vi "Ensure Parents are Expanded.vi"(8 "error in":errorcluster, 11 "Tree":refnum<vi>) -> (0 "error out":errorcluster)   [LabVIEW 2020]
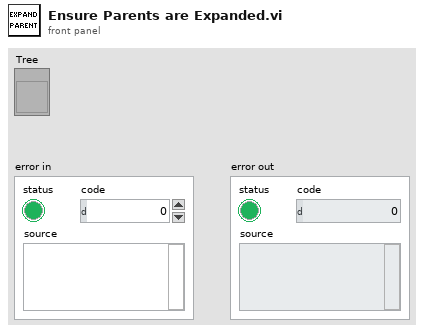
[diagram p1: front panel]
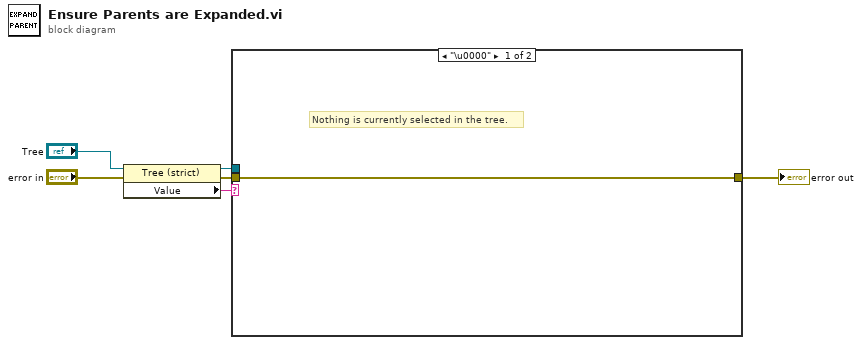
[diagram p0: block diagram]
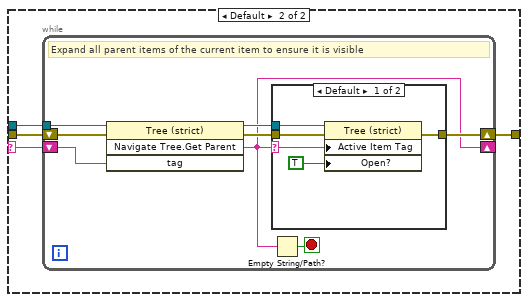
[diagram p2: hidden frame]
diagram:
  n1 = property class="Tree (strict)"(reference="Tree", error in="error in") -> (reference out=w1:refnum<vi>, error out=w5:errorcluster, "Value"=w2:string)
  n2 = case shown="\"\"" w2 {
    selector: w2 -> [_ w9]
    tunnel: w5 -> [w7 w11]
    tunnel: [w7 w10] -> w4
    tunnel: w1 -> [_ w8]
    frame "\u0000" {
      # "Nothing is currently selected in the tree."
    }
    frame Default {
      n3 = while {
        shift-right: [w13] -> _
        shift-left: w9 -> [w15]
        tunnel: w8 -> [w16]
        shift-right: [w17] -> w10
        shift-left: w11 -> [w19]
        stop <- w12 stop-if-true
        # "Expand all parent items of the current item to ensure it is visible"
        n4 = invoke class="Tree (strict)" method="Navigate Tree.Get Parent"(reference=w16, error in=w19, "tag"=w15) -> (reference out=w14:refnum<vi>, error out=w18:errorcluster, "Navigate Tree:Get Parent"=w13:string)  [unwired: 1 in, 1 out]
        n5 = case shown="Default" w13 {
          selector: w13 -> [w21 _]
          tunnel: w18 -> [w24 w25]
          tunnel: w14 -> [w22 _]
          tunnel: [w23 w25] -> w17
          frame Default {
            n6 = property class="Tree (strict)"(reference=w22, error in=w24, "Active Item Tag"=w21, "Open?"=TRUE ("Active Item:Open?")) -> (error out=w23:errorcluster)  [unwired: 1 out]
          }
          frame "" {
          }
        }
        n7 = Empty String/Path?(string/path=w13) -> (empty?=w12:bool)
      }
    }
  }
  "error out" <- w4
